vi "Lab2_2.vi"() -> ()   [LabVIEW 2021]
panel:
  out "bytes written":i32
  out "Recieved Value 2":dbl
  out "Recieved Value 1":dbl
  out "String that is Sent":string
  out "String that is Recieved":string
  in  "Send Value2":dbl
  in  "Send Value1":dbl
  in  "Send Button":bool
  in  "stop":bool
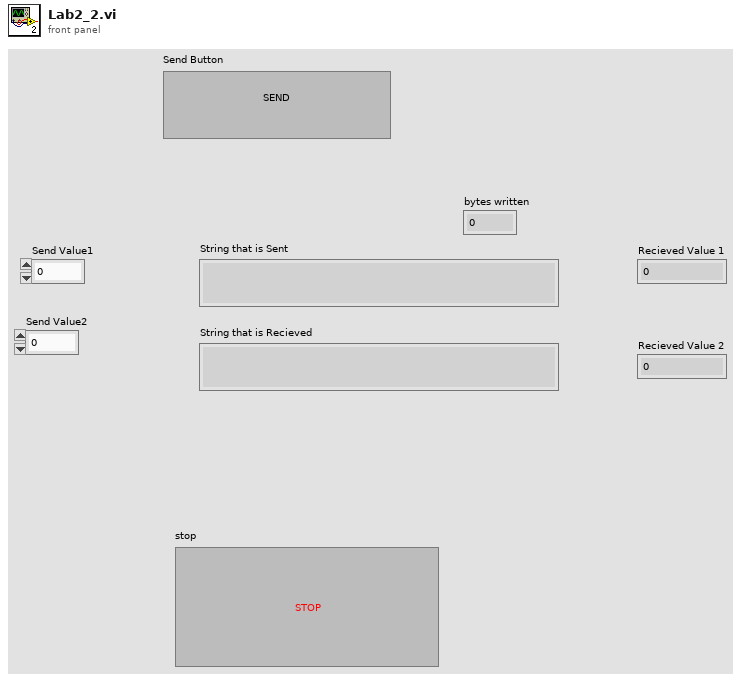
[diagram p1: front panel]
types:
  T1 = enum16{"Standard", "Buffered", "CRLF", "Immediate"}
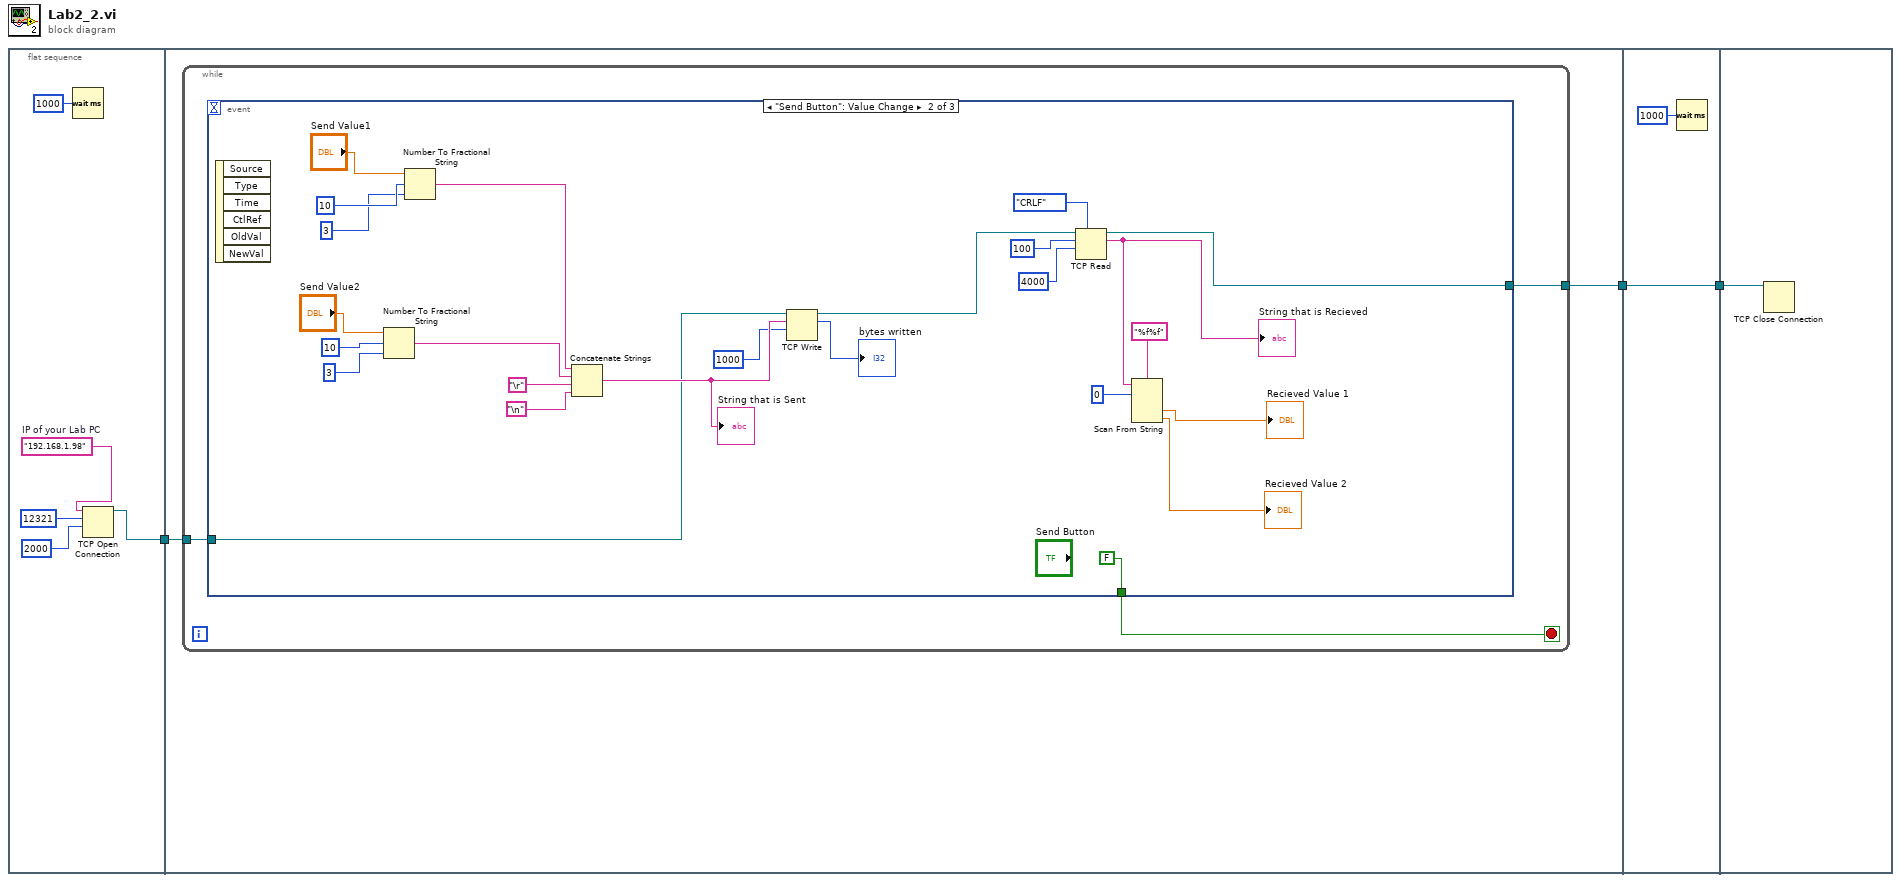
[diagram p0: block diagram]
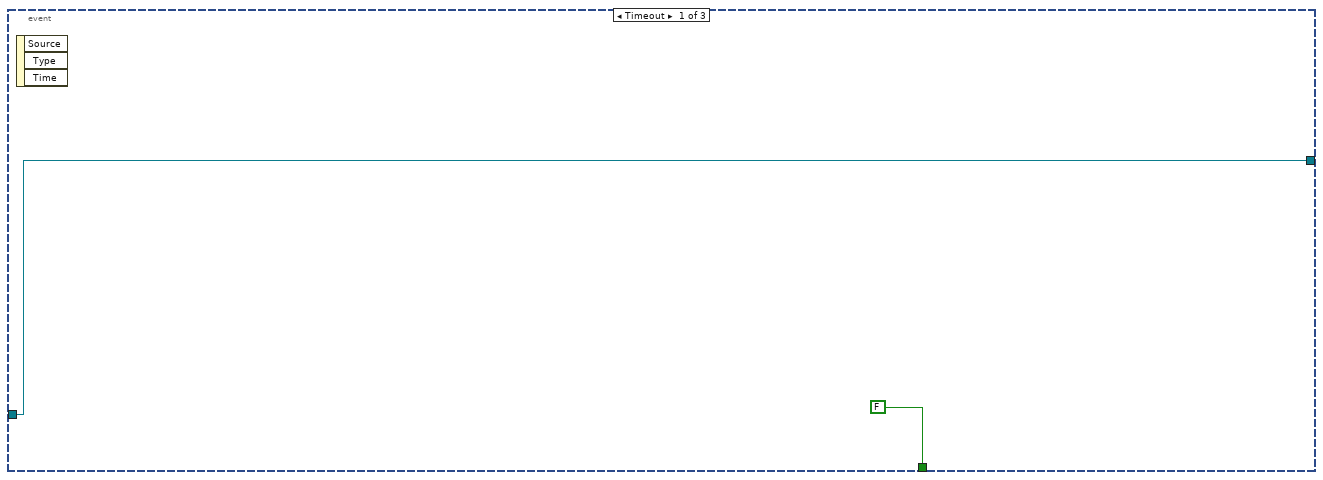
[diagram p2: hidden frame]
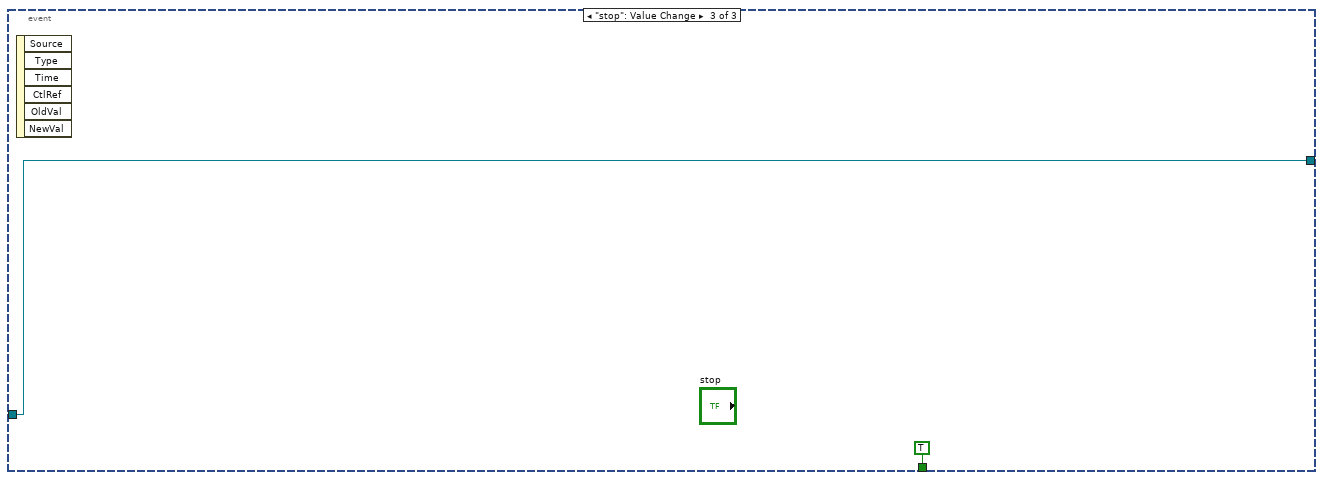
[diagram p3: hidden frame]
diagram:
  n1 = flat-sequence {
    tunnel: [w4] -> w3
    tunnel: w3 -> [w10]
    tunnel: [w9] -> w1
    tunnel: [w43] -> w2
    tunnel: w1 -> [w43]
    tunnel: w2 -> [w45]
    frame #0 {
      w7 = "192.168.1.98"  # IP of your Lab PC
      n2 = Wait (ms)(milliseconds to wait=u32 1000) -> ()  [unwired: 1 out]
      n3 = TCP Open Connection(address=w7, remote port or service name=u16 12321, timeout ms (60000)=2000) -> (connection ID=w4:refnum<k5>)  [unwired: 2 in, 1 out]
    }
    frame #1 {
      n4 = while {
        tunnel: w10 -> [w13]
        tunnel: [w12] -> w9
        stop <- w11 stop-if-true
        n5 = event shown="[1] \"Send Button\": Value Change" {
          selector: _ -> [_ _ _]
          dyn-events: _ -> [_ _ _]
          timeout: _ -> [_ _ _]
          tunnel: w13 -> [w15 w17 w41]
          tunnel: [w15 w27 w41] -> w12
          tunnel: [FALSE FALSE TRUE] -> w11
          event Timeout {
            n6 = event-data() -> ()  [unwired: 1 in, 3 out]
          }
          event "Send Button": Value Change {
            n7 = event-data() -> ()  [unwired: 1 in, 6 out]
            n8 = Number To Fractional String(number="Send Value2", width (-)=i16 10, precision (6)=i16 3) -> (F-format string=w33:string)  [unwired: 1 in]
            n9 = Number To Fractional String(number="Send Value1", width (-)=i16 10, precision (6)=i16 3) -> (F-format string=w34:string)  [unwired: 1 in]
            n10 = Concatenate Strings(w34, w33, "\r", "\n") -> (w30:string)
            "String that is Sent" <- w30
            n11 = TCP Write(connection ID=w17, data in=w30, 9:1000 ("timeout ms (25000)")) -> (connection ID out=w16:refnum<k5>, bytes written=→"bytes written":i32)  [unwired: 1 in, 1 out]
            n12 = TCP Read(connection ID=w16, bytes to read=100, 7:T1."CRLF" ("mode (standard)"), 9:4000 ("timeout ms (25000)")) -> (connection ID out=w27:refnum<k5>, data out=w26:string)  [unwired: 1 in, 1 out]
            "String that is Recieved" <- w26
            n13 = Scan From String "Scan From String"(format string="%f%f", input string=w26, initial scan location=u32 0) -> (output 1=→"Recieved Value 1":dbl, output 2=→"Recieved Value 2":dbl)  [unwired: 3 in, 3 out]
          }
          event "stop": Value Change {
            n14 = event-data() -> ()  [unwired: 1 in, 6 out]
          }
        }
      }
    }
    frame #2 {
      n15 = Wait (ms)(milliseconds to wait=u32 1000) -> ()  [unwired: 1 out]
    }
    frame #3 {
      n16 = TCP Close Connection(connection ID=w45) -> ()  [unwired: 2 in, 2 out]
    }
  }
